vi "Simple DMM SCAN PMPS 16V-15C - Loop.vi"() -> ()   [LabVIEW 2021]
uses:
  DMM SCAN PMPS 16V-15C/Typedefs/Scan configuration.ctl
  <instrlib>/niDMM/nidmm.llb/niDMM Resolution in Digits.ctl
  DMM SCAN PMPS 16V-15C/Typedefs/Formatted measurement.ctl
  DMM SCAN PMPS 16V-15C/Typedefs/Scan Resource Names.ctl
  DMM SCAN PMPS 16V-15C/DMM_Scan PXI Mux PXI Shunt 16V-15C.lvlib
panel:
  out "Total Scan Time (s)":dbl=0.1018724999994447 format="%#.3p"
  in  "Stop Button":bool
  out "error out":errorcluster
  out "Formatted Measurements":T1[](array[typedef])=[{"Channel"="ch16", "Switch Time"=0.03122810000058962, "Formatted Measurement"="1.00954mA (dc)", "Out of Range"=FALSE}, {"Channel"="ch17", "Switch Time"=0.016568299997743452, "Formatted Measurement"="10.0906uA (dc)", "Out of Range"=FALSE}, {"Channel"="ch18", "Switch Time"=0.01631730000008247, "Formatted Measurement"="1.00047mA (dc)", "Out of Range"=FALSE}, {"Channel"="ch1", "Switch Time"=0.015307000001484994, "Formatted Measurement"="9.99620V (dc)", "Out of Range"=FALSE}, {"Channel"="ch2", "Switch Time"=0.011196399998880224, "Formatted Measurement"="97.5985mV (dc)", "Out of Range"=FALSE}, {"Channel"="ch3", "Switch Time"=0.01125030000184779, "Formatted Measurement"="9.88503V (dc)", "Out of Range"=FALSE}] {"Switch Time" format="%#_3p"}
  in  "Scan Configuration":T2[](array[typedef])=[{"Channel"="ch16", "Resolution in Digits"=5.5, "Range and Function"=enum."DC 1 mA"}, {"Channel"="ch17", "Resolution in Digits"=5.5, "Range and Function"=enum."DC 100 uA"}, {"Channel"="ch18", "Resolution in Digits"=5.5, "Range and Function"=enum."DC 1 mA"}, {"Channel"="ch1", "Resolution in Digits"=5.5, "Range and Function"=enum."DC 10 V"}, {"Channel"="ch2", "Resolution in Digits"=5.5, "Range and Function"=enum."DC 100 mV"}, {"Channel"="ch3", "Resolution in Digits"=5.5, "Range and Function"=enum."DC 10 V"}] {"Resolution in Digits" items=["3 1/2"=3.5, "4 1/2"=4.5, "5 1/2"=5.5, "6 1/2"=6.5, "7 1/2"=7.5]}
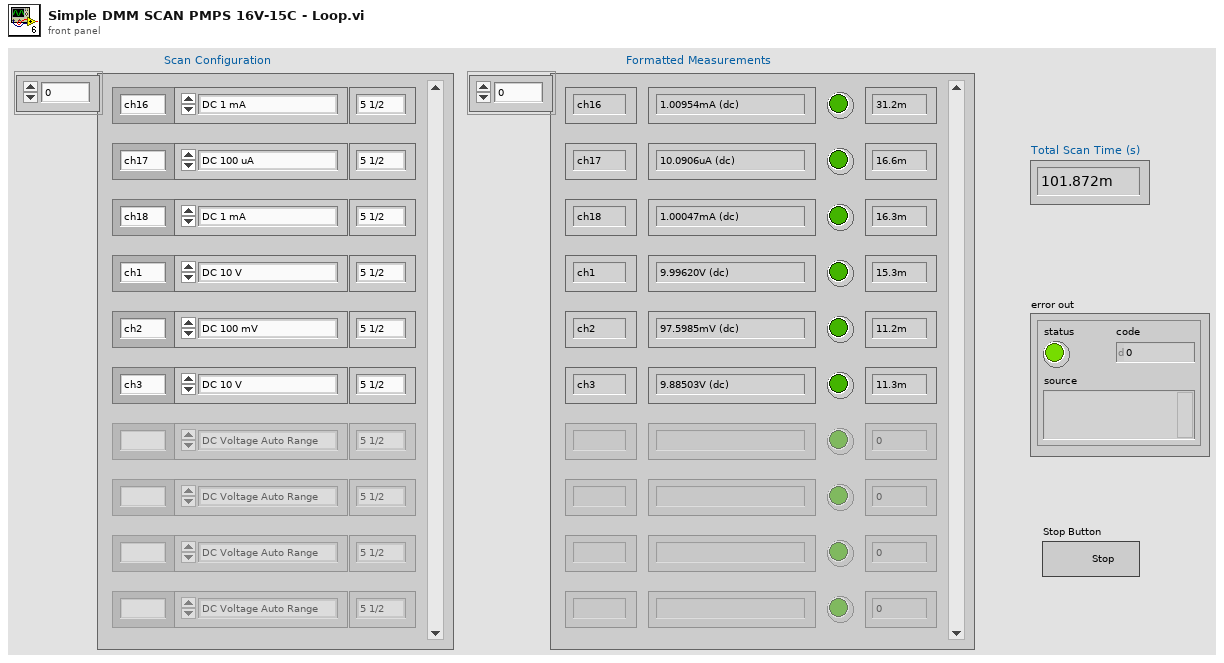
[diagram p1: front panel]
types:
  T1 = typedef "DMM_Scan PXI Mux PXI Shunt 16V-15C.lvlib/Formatted measurement.ctl" = cluster{"Channel":string, "Switch Time":dbl, "Formatted Measurement":string, "Out of Range":bool}
  T2 = typedef "DMM_Scan PXI Mux PXI Shunt 16V-15C.lvlib/Scan configuration.ctl" = cluster{"Channel":string, "Resolution in Digits":T3, "Range and Function":enum16{"DC Voltage Auto Range", "DC 100 mV", "DC 1 V ", "DC 10 V", "DC 100 V", "DC 300 V", " ", "AC Voltage Auto Range", "AC 50 mV", "AC 200 mV", "AC 500 mV", "AC 2 V", "AC 5 V", "AC 20 V", "AC 50 V", "AC 300 V", "  ", "DC Current Auto Range", "DC 1 uA", "DC 10 uA", "DC 100 uA", "DC 1 mA", "DC 10 mA", "DC 20 mA", "DC 100 mA", "DC 200 mA", "DC 1 A", "DC 3 A", "   ", "AC Current Auto Range", "AC 100 uA", "AC 1 mA", "AC 10 mA", "AC 100 mA", "AC 500 mA", "AC 1 A", "AC 3 A", "    ", "Resistance Auto Range", "Res 100 Ohm", "Res 1 kOhm", "Res 10 kOhm", "Res 100 kOhm", "Res 1 MOhm", "Res 10 MOhm", "Res 100 MOhm", "Res 5 GOhm", "     ", "Frequency AC Auto Range", "Freq AC 50 mV", "Freq AC 500 mV", "Freq AC 5 V", "Freq AC 50 V", "Freq AC 300 V", "      ", "Period AC Auto Range", "Period AC 50 mV", "Period AC 500 mV", "Period AC 5 V", "Period AC 50 V", "Period AC 300 V"}}
  T3 = typedef "niDMM Resolution in Digits.ctl" = dbl
  T4 = typedef "DMM_Scan PXI Mux PXI Shunt 16V-15C.lvlib/Scan Resource Names.ctl" = cluster{"DMM Resource Name":refnum<k15>, "MUX Resource Name":refnum<k15>, "Shunt Resource Name":refnum<k15>}
  T5 = typedef "DMM_Scan PXI Mux PXI Shunt 16V-15C.lvlib/Scan Resource Handles Out.ctl" = cluster{"DMM Handle":refnum<k15>, "MUX Handle":refnum<k15>, "Shunt Handle":refnum<k15>, "Close all Shunts?":bool}
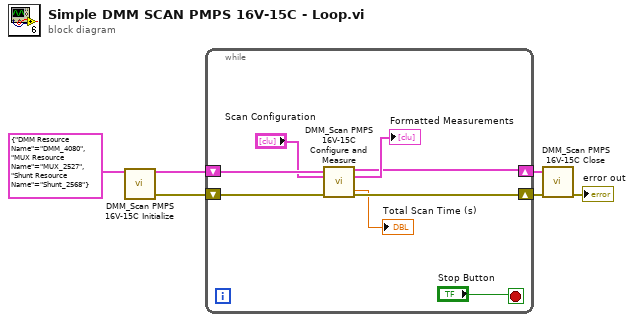
[diagram p0: block diagram]
diagram:
  n1 = call "DMM_Scan PMPS 16V-15C Initialize.vi"("Scan Resources Names"=T4 {"DMM Resource Name"="DMM_4080", "MUX Resource Name"="MUX_2527", "Shunt Resource Name"="Shunt_2568"} ("Scan resources Names")) -> ("Scan Resource Handles Out"=w4:T5, "error out"=w6:errorcluster)  [unwired: 12 in, 1 out]
  n2 = while {
    shift-right: [w13] -> w5
    shift-left: w6 -> [w14]
    shift-right: [w7] -> w1
    shift-left: w4 -> [w12]
    stop <- "Stop Button" stop-if-true
    n3 = call "DMM_Scan PMPS 16V-15C Configure and Measure.vi"("Scan Resources Handles In"=w12, "Scan Configuration"="Scan Configuration", "error in"=w14) -> ("Scan Resources Handles Out"=w7:T5, "Formatted Measurements"=→"Formatted Measurements":T1[], "Total Scan Time (s)"=→"Total Scan Time (s)":dbl, "error out"=w13:errorcluster)  [unwired: 7 in, 2 out]
  }
  n4 = call "DMM_Scan PMPS 16V-15C Close.vi"("Scan Resources Handles In"=w1, "error in"=w5) -> ("error out"=→"error out":errorcluster)  [unwired: 13 in]
